vi "Filter Logger.vi"() -> ()   [LabVIEW 2018]
panel:
  out "Waveform Chart":dynamicdata(graph)
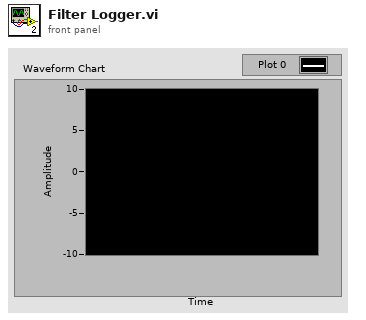
[diagram p1: front panel]
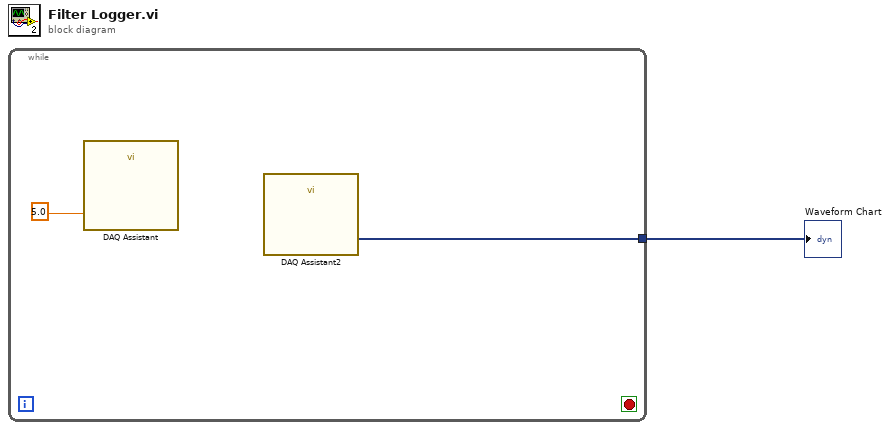
[diagram p0: block diagram]
diagram:
  n1 = while {
    tunnel: [w2] -> w1
    stop <- _ stop-if-true
    n2 = call "DAQ Assistant"("data"=5.0) -> ()  [unwired: 17 in, 2 out]
    n3 = call "DAQ Assistant2"() -> ("data"=w2:dynamicdata)  [unwired: 17 in, 2 out]
  }
  "Waveform Chart" <- w1
